vi "daxinf_to_tif.vi"(1 "String in":string, 2 "path in":path) -> ()   [LabVIEW 2011]
panel:
  out "No. of frames":i32
  out "Y pixel":i32
  out "X pixel":i32
  out "appended path 2":path
  out "length":i32
  out "concatenated string":string
  out "text":string
  out "appended path":path
  out "String out":string
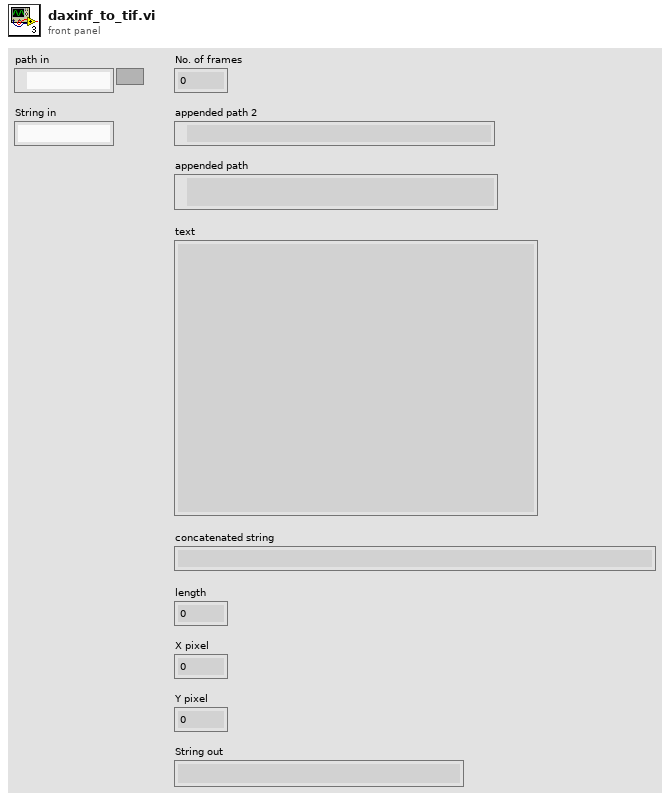
[diagram p1: front panel]
types:
  T1 = enum16{"big-endian, network order", "native, host order", "little-endian"}
  T2 = enum16{"open", "replace", "create", "open or create", "replace or create", "replace or create with confirmation"}
  T3 = cluster{cluster{i16, i16, i32}, "Number of tags":i16, cluster{i16, i16, i32, i32}, cluster{i16, i16, i32, "X pixel":i32}, cluster{i16, i16, i32, "Y pixel":i32}, cluster{i16, i16, i32, i32}, cluster{i16, i16, i32, i32}, cluster{i16, i16, i32, i32}, cluster{i16, i16, i32, i32}, cluster{i16, i16, i32, i32}, cluster{i16, i16, i32, i32}, cluster{i16, i16, i32, i32}, i32}
  T4 = cluster{"Number of tags":i16, cluster{i16, i16, i32, i32}, cluster{i16, i16, i32, "X pixel":i32}, cluster{i16, i16, i32, "Y pixel":i32}, cluster{i16, i16, i32, i32}, cluster{i16, i16, i32, i32}, cluster{i16, i16, i32, i32}, cluster{i16, i16, i32, i32}, cluster{i16, i16, i32, i32}, cluster{i16, i16, i32, i32}, cluster{i16, i16, i32, i32}, "y":i32}
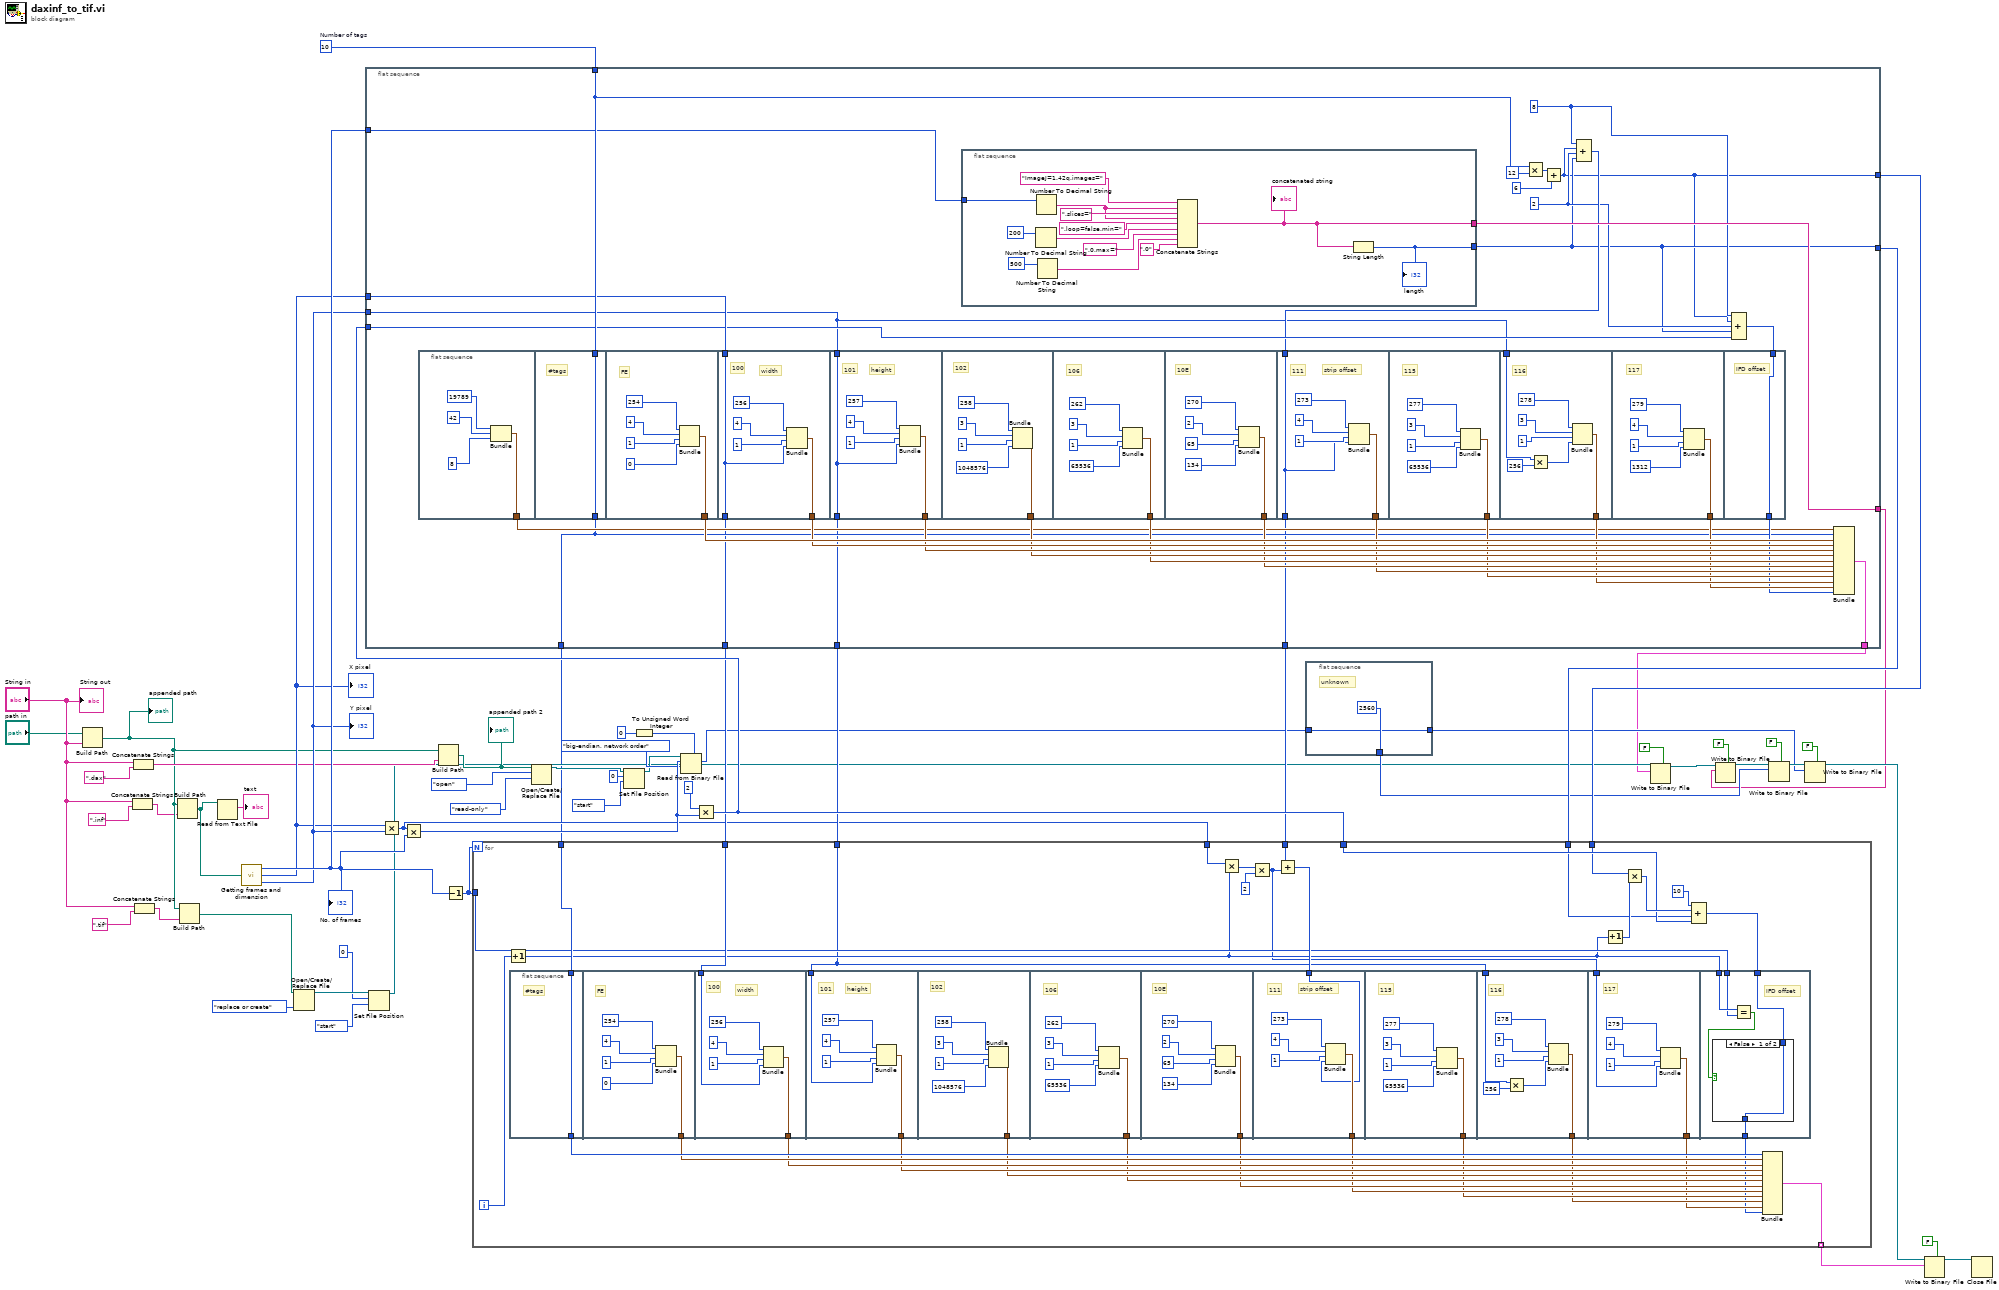
[diagram p0: block diagram]
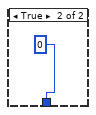
[diagram p2: hidden frame]
diagram:
  w16 = i16 10  # Number of tags
  n1 = Build Path(base path="path in", name or relative path="String in") -> (appended path=w26:path)
  "appended path" <- w26
  n2 = Concatenate Strings("String in", ".inf" ("pattern")) -> (w4:string)
  n3 = Concatenate Strings("String in", ".dax" ("pattern")) -> (w27:string)
  n4 = Concatenate Strings("String in", ".tif" ("pattern")) -> (w8:string)
  n5 = Build Path(base path=w26, name or relative path=w4) -> (appended path=w6:path)
  n6 = Build Path(base path=w26, name or relative path=w8) -> (appended path=w14:path)
  n7 = Read from Text File(file (use dialog)=w6) -> (text=→"text":string)  [unwired: 3 in, 3 out]
  n8 = call "Getting frames and dimension.vi"("Path"=w6) -> ("No. of frames"=w57:i32, "X pixel"=w48:i32, "Y pixel"=w49:i32)
  "X pixel" <- w48
  "Y pixel" <- w49
  "No. of frames" <- w57
  n9 = Open/Create/Replace File(file path (use dialog)=w14, operation (0:open)=T2."replace or create") -> (refnum out=w13:refnum<file>)  [unwired: 4 in, 2 out]
  n10 = flat-sequence {
    tunnel: [w78] -> w15
    tunnel: w16 -> [w77]
    tunnel: [w75] -> w18
    tunnel: [w74] -> w22
    tunnel: [w73] -> w46
    tunnel: w48 -> [w72]
    tunnel: w49 -> [w59]
    tunnel: [w71] -> w50
    tunnel: [w70] -> w51
    tunnel: w55 -> [w69]
    tunnel: [w61] -> w56
    tunnel: w57 -> [w67]
    tunnel: [w60] -> w58
    frame #0 {
      w62 = 2 ("x")
      w63 = 8 ("x")
      n11 = flat-sequence {
        tunnel: [w104] -> w79
        tunnel: [w108] -> w78
        tunnel: w77 -> [w108]
        tunnel: [w109] -> w90
        tunnel: [w115] -> w89
        tunnel: w72 -> [w114]
        tunnel: [w114] -> w71
        tunnel: [w120] -> w88
        tunnel: w59 -> [w119]
        tunnel: [w119] -> w70
        tunnel: [w125] -> w87
        tunnel: [w129] -> w86
        tunnel: [w134] -> w85
        tunnel: [w140] -> w84
        tunnel: w64 -> [w139]
        tunnel: [w139] -> w73
        tunnel: [w144] -> w83
        tunnel: [w153] -> w82
        tunnel: w59 -> [w151]
        tunnel: [w156] -> w81
        tunnel: [w161] -> w80
        tunnel: w68 -> [w161]
        frame #0 {
          n12 = Bundle(i16 19789, i16 42, 8) -> (w104:cluster{i16, i16, i32})  [unwired: 1 in]
        }
        frame #1 {
          # "#tags"
        }
        frame #2 {
          # "FE"
          n13 = Bundle(i16 254, i16 4, 1, 0) -> (w109:cluster{i16, i16, i32, i32})  [unwired: 1 in]
        }
        frame #3 {
          # "width"
          # "100"
          n14 = Bundle(i16 256, i16 4, 1, "X pixel"=w114) -> (w115:cluster{i16, i16, i32, "X pixel":i32})  [unwired: 1 in]
        }
        frame #4 {
          # "height"
          # "101"
          n15 = Bundle(i16 257, i16 4, 1, "Y pixel"=w119) -> (w120:cluster{i16, i16, i32, "Y pixel":i32})  [unwired: 1 in]
        }
        frame #5 {
          # "102"
          n16 = Bundle(i16 258, i16 3, 1, 1048576) -> (w125:cluster{i16, i16, i32, i32})  [unwired: 1 in]
        }
        frame #6 {
          # "106"
          n17 = Bundle(i16 262, i16 3, 1, 65536) -> (w129:cluster{i16, i16, i32, i32})  [unwired: 1 in]
        }
        frame #7 {
          # "10E"
          n18 = Bundle(i16 270, i16 2, 65, 134) -> (w134:cluster{i16, i16, i32, i32})  [unwired: 1 in]
        }
        frame #8 {
          # "strip offset"
          # "111"
          n19 = Bundle(i16 273, i16 4, 1, w139) -> (w140:cluster{i16, i16, i32, i32})  [unwired: 1 in]
        }
        frame #9 {
          # "115"
          n20 = Bundle(i16 277, i16 3, 1, 65536) -> (w144:cluster{i16, i16, i32, i32})  [unwired: 1 in]
        }
        frame #10 {
          # "116"
          n21 = Multiply(x=w151, y=256) -> (x*y=w150:i32)
          n22 = Bundle(i16 278, i16 3, 1, w150) -> (w153:cluster{i16, i16, i32, i32})  [unwired: 1 in]
        }
        frame #11 {
          # "117"
          n23 = Bundle(i16 279, i16 4, 1, 1312) -> (w156:cluster{i16, i16, i32, i32})  [unwired: 1 in]
        }
        frame #12 {
          # "IFD offset"
        }
      }
      n24 = flat-sequence {
        tunnel: [w92] -> w74
        tunnel: [w93] -> w61
        tunnel: w67 -> [w91]
        frame #0 {
          n25 = Number To Decimal String(number=200) -> (decimal integer string=w97:string)  [unwired: 1 in]
          n26 = Number To Decimal String(number=w91) -> (decimal integer string=w99:string)  [unwired: 1 in]
          n27 = Number To Decimal String(number=500) -> (decimal integer string=w95:string)  [unwired: 1 in]
          n28 = Concatenate Strings("ImageJ=1.42q.images=" ("string"), w99, ".slices=" ("string"), w99, ".loop=false.min=" ("string"), w97, ".0.max=" ("string"), w95, ".0" ("string")) -> (w92:string)
          "concatenated string" <- w92
          n29 = String Length(string=w92) -> (length=w93:i32)
          "length" <- w93
        }
      }
      n30 = Multiply(x=w77, y=12) -> (x*y=w66:i32)
      n31 = Add(x=w66, y=6 ("x")) -> (x+y=w60:i32)
      n32 = Compound Arithmetic op=ADD(w63, w60, w62, w61) -> (w64:i32)
      n33 = Compound Arithmetic op=ADD(w63, w60, w62, w61, w69) -> (w68:i32)
      n34 = Bundle(w79, "Number of tags"=w78, w90, w89, w88, w87, w86, w85, w84, w83, w82, w81, w80) -> (w75:T3)  [unwired: 1 in]
    }
  }
  n35 = Set File Position(offset (in bytes) (0)=i64 0, refnum=w13, from (0:start)=enum16{"start", "end", "current"}."start") -> (refnum out=w20:refnum<file>)  [unwired: 1 in, 1 out]
  n36 = Multiply(x=w48, y=w49) -> (x*y=w47:i32)
  n37 = Multiply(x=w47, y=w57) -> (x*y=w54:i32)
  n38 = Build Path(base path=w26, name or relative path=w27) -> (appended path=w34:path)
  "appended path 2" <- w34
  n39 = Decrement(x=w57) -> (x-1=w52:i32)
  n40 = Open/Create/Replace File(file path (use dialog)=w34, operation (0:open)=T2."open", access (0:read/write)=enum16{"read/write", "read-only", "write-only"}."read-only") -> (refnum out=w35:refnum<file>)  [unwired: 3 in, 2 out]
  n41 = Set File Position(offset (in bytes) (0)=i64 0, refnum=w35, from (0:start)=enum16{"start", "end", "current"}."start") -> (refnum out=w36:refnum<file>)  [unwired: 1 in, 1 out]
  n42 = To Unsigned Word Integer(number=u16 0) -> (unsigned 16bit integer=w41:u16)
  n43 = Read from Binary File(5:w41, 9:T1."big-endian, network order" ("byte order (0:big-endian, network order)"), 10:w54, 11:w36) -> (2:w28:u16[])  [unwired: 2 in, 3 out]
  n44 = Multiply(x=2, y=w54) -> (x*y=w55:i32)
  n45 = for {
    N: w52 -> [_]
    tunnel: w15 -> [w181]
    tunnel: [w180] -> w45 mode=indexing
    tunnel: w46 -> [w178]
    tunnel: w47 -> [w173]
    tunnel: w50 -> [w176]
    tunnel: w51 -> [w163]
    tunnel: w52 -> [w174]
    tunnel: w55 -> [w168]
    tunnel: w56 -> [w166]
    tunnel: w58 -> [w164]
    i -> [w172]
    n46 = Increment(x=w172) -> (x+1=w165:i32)
    n47 = flat-sequence {
      tunnel: [w194] -> w193
      tunnel: w181 -> [w194]
      tunnel: [w195] -> w192
      tunnel: [w201] -> w191
      tunnel: w176 -> [w200]
      tunnel: [w206] -> w190
      tunnel: w163 -> [w205]
      tunnel: [w211] -> w189
      tunnel: [w215] -> w188
      tunnel: [w220] -> w187
      tunnel: [w226] -> w186
      tunnel: w177 -> [w225]
      tunnel: [w230] -> w185
      tunnel: [w238] -> w184
      tunnel: w163 -> [w237]
      tunnel: [w243] -> w183
      tunnel: w162 -> [w242]
      tunnel: [w248] -> w182
      tunnel: w165 -> [w251]
      tunnel: w174 -> [w250]
      tunnel: w167 -> [w247]
      frame #0 {
        # "#tags"
      }
      frame #1 {
        # "FE"
        n48 = Bundle(i16 254, i16 4, 1, 0) -> (w195:cluster{i16, i16, i32, i32})  [unwired: 1 in]
      }
      frame #2 {
        # "width"
        # "100"
        n49 = Bundle(i16 256, i16 4, 1, "X pixel"=w200) -> (w201:cluster{i16, i16, i32, "X pixel":i32})  [unwired: 1 in]
      }
      frame #3 {
        # "height"
        # "101"
        n50 = Bundle(i16 257, i16 4, 1, "Y pixel"=w205) -> (w206:cluster{i16, i16, i32, "Y pixel":i32})  [unwired: 1 in]
      }
      frame #4 {
        # "102"
        n51 = Bundle(i16 258, i16 3, 1, 1048576) -> (w211:cluster{i16, i16, i32, i32})  [unwired: 1 in]
      }
      frame #5 {
        # "106"
        n52 = Bundle(i16 262, i16 3, 1, 65536) -> (w215:cluster{i16, i16, i32, i32})  [unwired: 1 in]
      }
      frame #6 {
        # "10E"
        n53 = Bundle(i16 270, i16 2, 65, 134) -> (w220:cluster{i16, i16, i32, i32})  [unwired: 1 in]
      }
      frame #7 {
        # "strip offset"
        # "111"
        n54 = Bundle(i16 273, i16 4, 1, w225) -> (w226:cluster{i16, i16, i32, i32})  [unwired: 1 in]
      }
      frame #8 {
        # "115"
        n55 = Bundle(i16 277, i16 3, 1, 65536) -> (w230:cluster{i16, i16, i32, i32})  [unwired: 1 in]
      }
      frame #9 {
        # "116"
        n56 = Multiply(x=w237, y=256) -> (x*y=w236:i32)
        n57 = Bundle(i16 278, i16 3, 1, w236) -> (w238:cluster{i16, i16, i32, i32})  [unwired: 1 in]
      }
      frame #10 {
        # "117"
        n58 = Bundle(i16 279, i16 4, 1, w242) -> (w243:cluster{i16, i16, i32, i32})  [unwired: 1 in]
      }
      frame #11 {
        # "IFD offset"
        n59 = Equal?(x=w251, y=w250) -> (x = y?=w249:bool)
        n60 = case shown="False" w249 {
          tunnel: [w252 0 ("y")] -> w248
          tunnel: w247 -> [w252 _]
          frame False {
          }
          frame True {
          }
        }
      }
    }
    n61 = Multiply(x=w173, y=w165) -> (x*y=w175:i32)
    n62 = Multiply(x=w175, y=2) -> (x*y=w162:i32)
    n63 = Add(x=w178, y=w162) -> (x+y=w177:i32)
    n64 = Increment(x=w165) -> (x+1=w171:i32)
    n65 = Multiply(x=w164, y=w171) -> (x*y=w170:i32)
    n66 = Compound Arithmetic op=ADD(10 ("x"), w170, w166, w168) -> (w167:i32)
    n67 = Bundle("Number of tags"=w193, w192, w191, w190, w189, w188, w187, w186, w185, w184, w183, "y"=w182) -> (w180:T4)  [unwired: 1 in]
  }
  n68 = flat-sequence {
    tunnel: [i16 2560] -> w25
    tunnel: w28 -> [w254]
    tunnel: [w254] -> w29
    frame #0 {
      # "unknown"
    }
  }
  n69 = Write to Binary File(file (use dialog)=w20, data=w18, 5:FALSE ("prepend array or string size? (T)")) -> (refnum out=w19:refnum<file>)  [unwired: 3 in, 2 out]
  n70 = Write to Binary File(file (use dialog)=w19, data=w22, 5:FALSE ("prepend array or string size? (T)")) -> (refnum out=w24:refnum<file>)  [unwired: 3 in, 2 out]
  n71 = Write to Binary File(file (use dialog)=w24, data=w25, 5:FALSE ("prepend array or string size? (T)")) -> (refnum out=w30:refnum<file>)  [unwired: 3 in, 2 out]
  n72 = Write to Binary File(file (use dialog)=w30, data=w29, 5:FALSE ("prepend array or string size? (T)")) -> (refnum out=w43:refnum<file>)  [unwired: 3 in, 2 out]
  n73 = Write to Binary File(file (use dialog)=w43, data=w45, 5:FALSE ("prepend array or string size? (T)")) -> (refnum out=w44:refnum<file>)  [unwired: 3 in, 2 out]
  n74 = Close File(refnum=w44) -> ()  [unwired: 1 in, 2 out]
  "String out" <- "String in"
